vi "Write Path.vi"(8 "error in (no error)":errorcluster, 10 "Path":path, 11 "Txt in":refnum<class "Txt.lvclass">) -> (0 "error out":errorcluster, 3 "Txt out":refnum<class "Txt.lvclass">)   [LabVIEW 2020, in "Txt.lvlib" / "Txt.lvclass"]
uses:
  Txt.lvclass
  Txt.lvclass/Txt.ctl
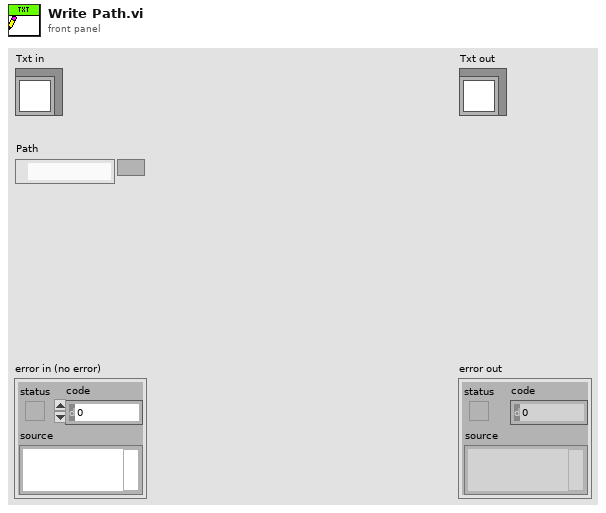
[diagram p1: front panel]
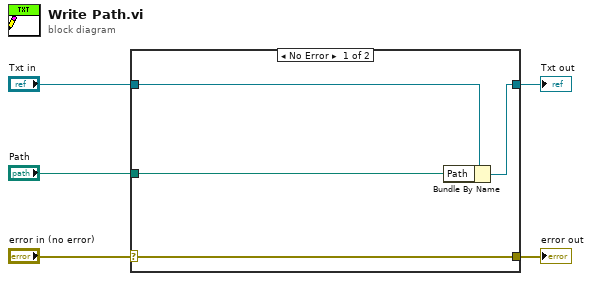
[diagram p0: block diagram]
diagram:
  n1 = case shown="No Error" "error in (no error)" {
    selector: "error in (no error)" -> [w9 w10]
    tunnel: [w9 w10] -> w4
    tunnel: [w7 w11] -> w2
    tunnel: "Txt in" -> [w8 w11]
    tunnel: "Path" -> [w6 _]
    frame No Error {
      n2 = Bundle By Name(cluster=w8, "Path"=w6) -> (w7:refnum<class "Txt.lvclass">)
    }
    frame Error {
    }
  }
  "error out" <- w4
  "Txt out" <- w2
